vi "FTW-ActorConnector-Test.vi"() -> ()   [LabVIEW 2013]
uses:
  Actor/src/Connector/FTW-ActorConnector.lvclass
panel:
  out "Avg Roundtrip Time":dbl format="%#_6p"
  in  "Messages":i32=1
  out "Timed out?":bool
  out "Ping Response":string
  in  "Connection":string(combo)="lvq://someLVQconnection"
  out "error out":errorcluster
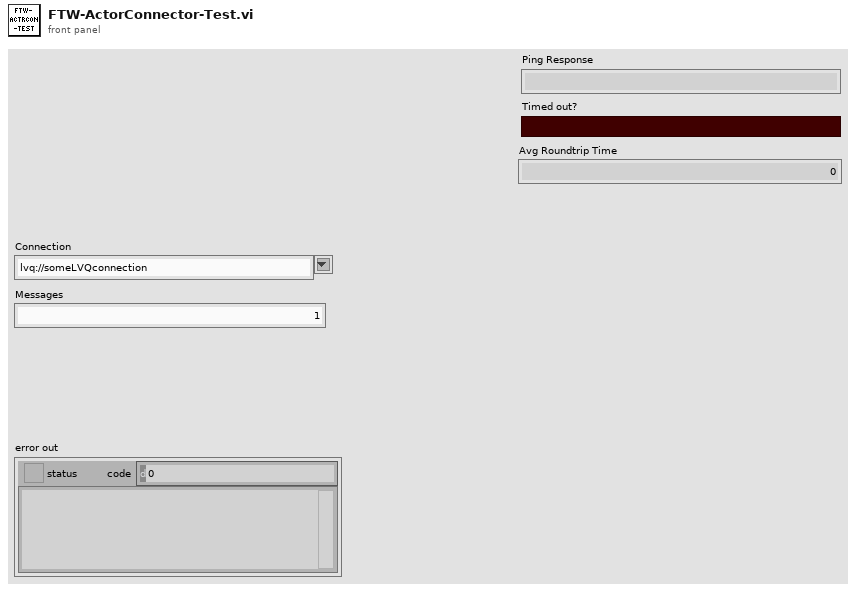
[diagram p1: front panel]
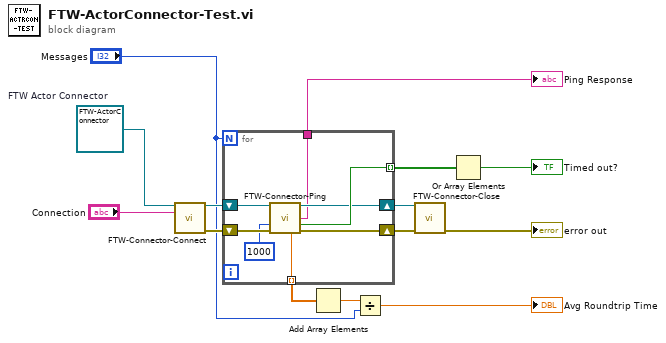
[diagram p0: block diagram]
diagram:
  w10 = refnum<class "FTW-ActorConnector.lvclass"> refnum  # FTW Actor Connector
  n1 = call-dynamic "FTW-Connector-Connect.vi"("FTW Actor Connector Type"=w10, "Instance Inbox Address"="Connection") -> ("FTW Actor Connector"=w9:refnum<class "FTW-ActorConnector.lvclass">, "error out"=w8:errorcluster)  [unwired: 12 in]
  n2 = for {
    N: "Messages" -> [_]
    tunnel: [w16] -> w13
    tunnel: [w22] -> w11 mode=indexing
    shift-right: [w18] -> w6
    shift-left: w8 -> [w20]
    shift-right: [w19] -> w7
    shift-left: w9 -> [w21]
    tunnel: [w15] -> w4 mode=indexing
    n3 = call "FTW-Connector-Ping.vi"("FTW Actor Connector"=w21, "Timeout"=1000, "error in"=w20) -> ("FTW Actor Connector out"=w19:refnum<class "FTW-ActorConnector.lvclass">, "Response Body"=w16:string, "Timed out?"=w22:bool, "Roundtrip Time"=w15:dbl, "error out"=w18:errorcluster)  [unwired: 8 in]
  }
  "Ping Response" <- w13
  n4 = Add Array Elements(numeric array=w4) -> (sum=w3:dbl)
  n5 = Divide(x=w3, y="Messages") -> (x/y=→"Avg Roundtrip Time":dbl)
  n6 = call-dynamic "FTW-Connector-Close.vi"("FTW Actor Connector"=w7, "error in"=w6) -> ("error out"=→"error out":errorcluster)  [unwired: 13 in]
  n7 = Or Array Elements(Boolean array=w11) -> (logical OR=→"Timed out?":bool)
